vi "Example WhileLoop ForLoop CaseStructure.vi"(8 "Error In":errorcluster, 11 "Boolean":bool) -> (0 "Error Out":errorcluster)   [LabVIEW 2014]
doc: "Testing VI contains WhileLoop and som operations inside and some other constants and functions for numbers used inside WhileLoop. Just for example parsing."
uses:
  <vilib>/measure/NI_MABase.lvlib
panel:
  out "appended array":waveform(dbl)[](array[waveform])
  out "signal out 3":waveform(dbl)
  out "String":string
  in  "stop":bool
  out "signal out 2":waveform(dbl)
  out "signal out":waveform(dbl)
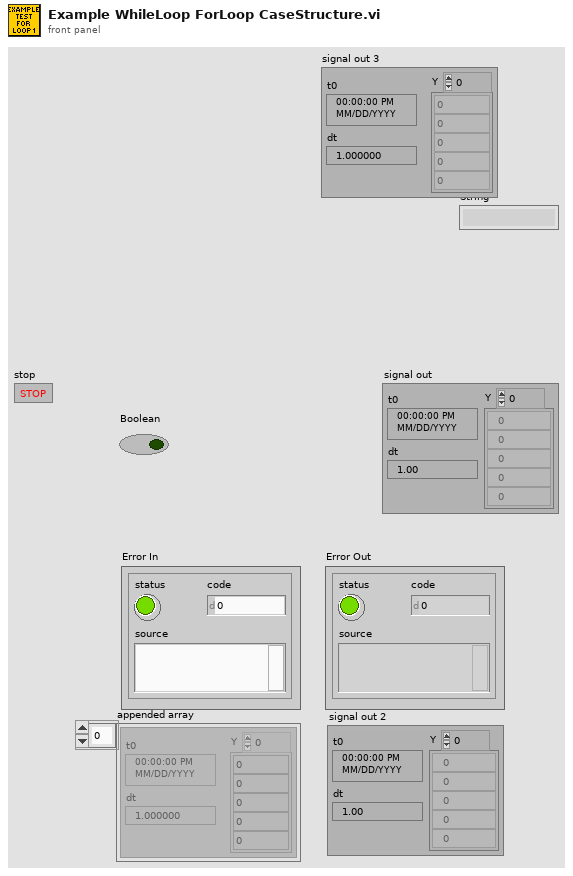
[diagram p1: front panel]
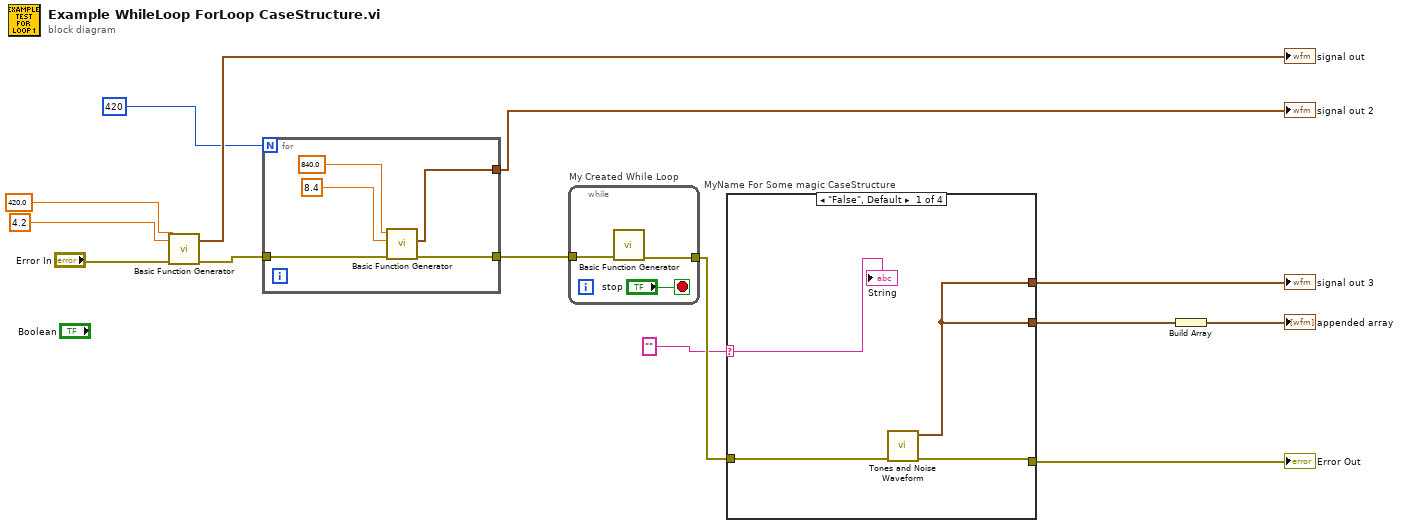
[diagram p0: block diagram]
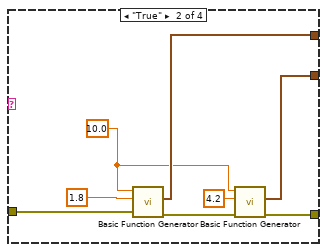
[diagram p2: hidden frame]
diagram:
  n1 = call <vilib>:"Basic Function Generator.vi"("error in (no error)"="Error In", "amplitude"=4.2, "frequency"=420.0) -> ("error out"=w13:errorcluster, "signal out"=→"signal out":waveform(dbl))  [unwired: 6 in, 1 out]
  n2 = for {
    N: 420 -> [_]
    tunnel: [w15] -> w9
    tunnel: w13 -> [w19]
    tunnel: [w18] -> w7
    n3 = call <vilib>:"Basic Function Generator.vi"("error in (no error)"=w19, "amplitude"=8.4, "frequency"=840.0) -> ("error out"=w18:errorcluster, "signal out"=w15:waveform(dbl))  [unwired: 6 in, 1 out]
  }
  "signal out 2" <- w9
  n4 = while "My Created While Loop" {
    tunnel: w7 -> [w21]
    tunnel: [w20] -> w3
    stop <- "stop" stop-if-true
    n5 = call <vilib>:"Basic Function Generator.vi"("error in (no error)"=w21) -> ("error out"=w20:errorcluster)  [unwired: 8 in, 2 out]
  }
  n6 = case "MyName For Some magic CaseStructure" shown="\"False\", Default" "" {
    selector: "" -> [w23 _ _ _]
    tunnel: w3 -> [w26 w34 w35 w36]
    tunnel: [w25 w32 w35 w36] -> w2
    tunnel: [w24 w29 _ _] -> w6
    tunnel: [w24 w28 _ _] -> w5
    frame "False", Default {
      n7 = call <vilib>:"Tones and Noise Waveform.vi"("error in (no error)"=w26) -> ("error out"=w25:errorcluster, "signal out"=w24:waveform(dbl))  [unwired: 9 in]
      "String" <- w23
    }
    frame "True" {
      w27 = 10.0 ("frequency")
      n8 = call <vilib>:"Basic Function Generator.vi"("error in (no error)"=w34, "amplitude"=1.8, "frequency"=w27) -> ("error out"=w33:errorcluster, "signal out"=w29:waveform(dbl))  [unwired: 6 in, 1 out]
      n9 = call <vilib>:"Basic Function Generator.vi"("error in (no error)"=w33, "amplitude"=4.2, "frequency"=w27) -> ("error out"=w32:errorcluster, "signal out"=w28:waveform(dbl))  [unwired: 6 in, 1 out]
    }
    frame "hello world" {
    }
    frame "some title" {
    }
  }
  "Error Out" <- w2
  "signal out 3" <- w6
  n10 = Build Array(w5) -> (→"appended array":waveform(dbl)[])
